vi "Parse.vi"(11 "Algo":string) -> (3 "output cluster":T1={"queue"=refnum, "error"={"status"=FALSE, "code"=0, "source"=""}, "Step"={"Name"="", "Timeout"=0.0}, "Algorythm"=[{"Name"="Init", "Timeout"=0.0}]})   [LabVIEW 2023, in "SFC.lvlib"]
uses:
  SFC.lvlib
  TypeDef/Control TypeDef.ctl
  TypeDef/Step TypeDef.ctl
panel:
  out "Args":dbl[](array[numeric])
  out "Steps":string[](array[string])
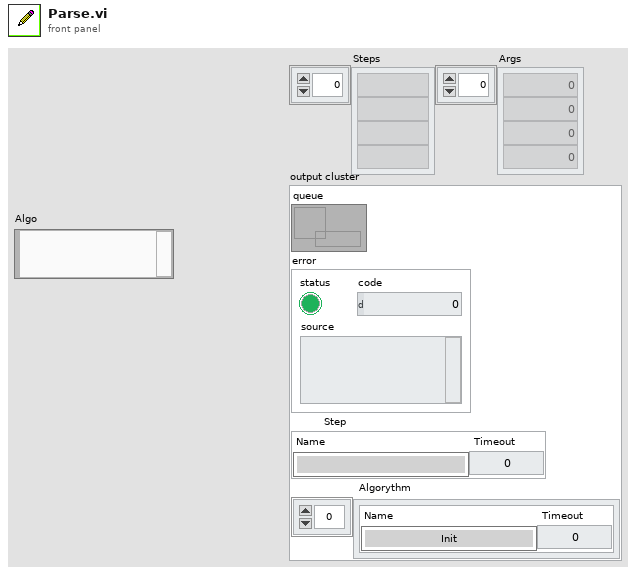
[diagram p1: front panel]
types:
  T1 = typedef "SFC.lvlib/Control TypeDef.ctl" = cluster{"queue":refnum<queue>, "error":errorcluster, "Step":T2, "Algorythm":T2[]}
  T2 = typedef "SFC.lvlib/Step TypeDef.ctl" = cluster{"Name":string, "Timeout":dbl}
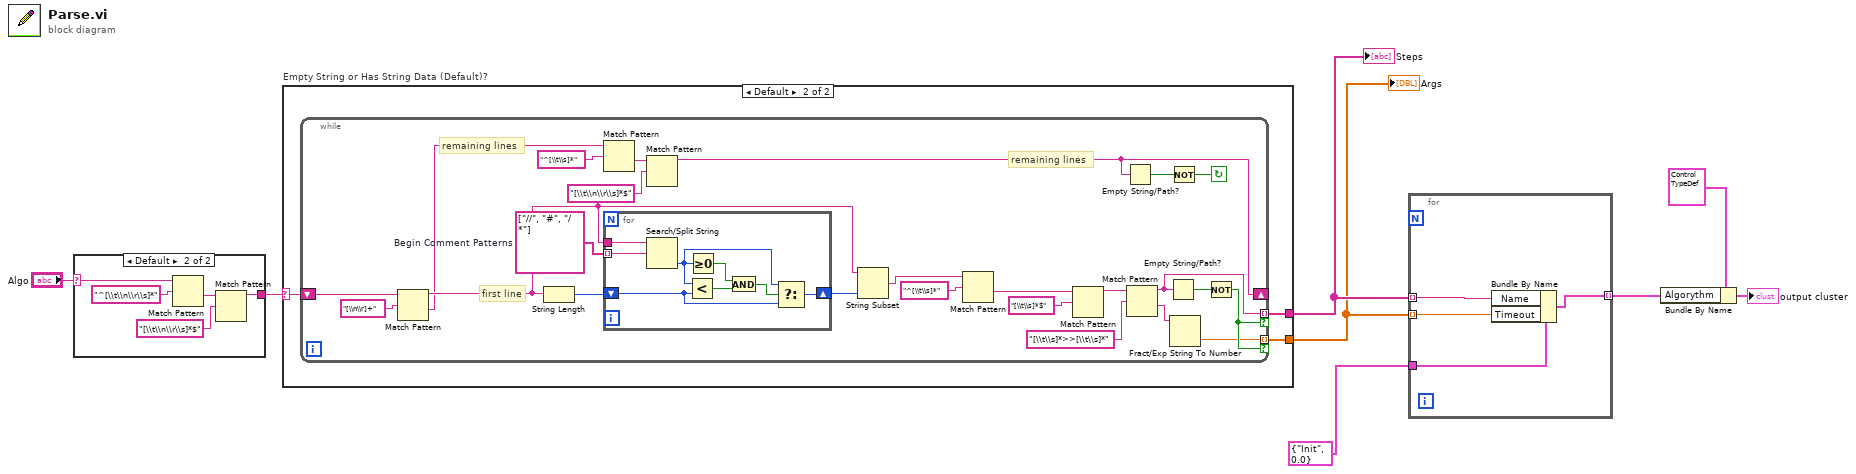
[diagram p0: block diagram]
diagram:
  n1 = case shown="Default" "Algo" {
    selector: "Algo" -> [_ w9]
    tunnel: [_ w10] -> w7
    frame "" {
    }
    frame Default {
      n2 = Match Pattern(string=w9, regular expression="^[\\t\\n\\r\\s]*") -> (after substring=w12:string)  [unwired: 1 in, 3 out]
      n3 = Match Pattern(string=w12, regular expression="[\\t\\n\\r\\s]*$") -> (before substring=w10:string)  [unwired: 1 in, 3 out]
    }
  }
  n4 = case "Empty String or Has String Data (Default)?" shown="Default" w7 {
    selector: w7 -> [_ w14]
    tunnel: [_ w16] -> w4
    tunnel: [_ w15] -> w3
    frame "" {
      # "Do Nothing if Empty String"
      # "<< Wiring into the Case Selector is much more performant than using \"Empty String/Path?\" primitive"
    }
    frame Default {
      n5 = while "While current line is a comment and there are more lines to process" {
        tunnel: [w21] -> w16 mode=indexing if=w19
        tunnel: [w17] -> w15 mode=indexing if=w19
        shift-right: [w39] -> _
        shift-left: w14 -> [w37]
        stop <- w22 continue-if-true
        w36 = string[] ["//", "#", "/*"]  # Begin Comment Patterns
        # "remaining lines"
        # "remaining lines"
        # "first line"
        n6 = Match Pattern(string=w37, regular expression="[\\n\\r]+") -> (before substring=w34:string, after substring=w27:string)  [unwired: 1 in, 2 out]
        n7 = String Length(string=w34) -> (length=w24:i32)
        n8 = Match Pattern(string=w27, regular expression="^[\\t\\s]*") -> (after substring=w26:string)  [unwired: 1 in, 3 out]
        n9 = for {
          tunnel: w36 -> [w45] mode=indexing
          shift-right: [w47] -> w23
          shift-left: w24 -> [w48]
          tunnel: w34 -> [w46]
          n10 = Search/Split String(string=w46, search string/char (-)=w45) -> (offset of match=w44:i32)  [unwired: 1 in, 2 out]
          n11 = Less?(x=w44, y=w48) -> (x < y?=w42:bool)
          n12 = Greater Or Equal To 0?(x=w44) -> (x >= 0?=w43:bool)
          n13 = And(x=w43, y=w42) -> (x .and. y?=w41:bool)
          n14 = Select(t=w44, s=w41, f=w48) -> (s? t:f=w47:i32)
        }
        n15 = Match Pattern(string=w26, regular expression="[\\t\\n\\r\\s]*$") -> (before substring=w39:string)  [unwired: 1 in, 3 out]
        n16 = String Subset(string=w34, length (rest)=w23) -> (substring=w35:string)  [unwired: 1 in]
        n17 = Match Pattern(string=w35, regular expression="^[\\t\\s]*") -> (after substring=w25:string)  [unwired: 1 in, 3 out]
        n18 = Match Pattern(string=w25, regular expression="[\\t\\s]*$") -> (before substring=w29:string)  [unwired: 1 in, 3 out]
        n19 = Empty String/Path?(string/path=w39) -> (empty?=w40:bool)
        n20 = Match Pattern(string=w29, regular expression="[\\t\\s]*>>[\\t\\s]*") -> (before substring=w21:string, after substring=w18:string)  [unwired: 1 in, 2 out]
        n21 = Empty String/Path?(string/path=w21) -> (empty?=w20:bool)
        n22 = Not(x=w40) -> (.not. x?=w22:bool)
        n23 = Fract/Exp String To Number(string=w18) -> (number=w17:dbl)  [unwired: 3 in, 1 out]
        n24 = Not(x=w20) -> (.not. x?=w19:bool)
      }
    }
  }
  "Steps" <- w4
  "Args" <- w3
  n25 = for {
    tunnel: T2 {"Name"="Init", "Timeout"=0.0} ("Step") -> [w52]
    tunnel: [w49] -> w5 mode=indexing
    tunnel: w4 -> [w51] mode=indexing
    tunnel: w3 -> [w50] mode=indexing
    n26 = Bundle By Name(cluster=w52, "Name"=w51, "Timeout"=w50) -> (w49:T2)
  }
  n27 = Bundle By Name(cluster=T1 {"queue"=refnum, "error"={"status"=FALSE, "code"=0, "source"=""}, "Step"={"Name"="", "Timeout"=0.0}, "Algorythm"=[{"Name"="Start", "Timeout"=3.0}, {"Name"="Work", "Timeout"=2.0}, {"Name"="Finish", "Timeout"=1.0}]} ("input cluster"), "Algorythm"=w5) -> (→"output cluster":T1)
